vi "Teleop.vi"(10 "Match Info":T1={"Autonomous Elapsed Seconds"=0.0, "TeleOp Elapsed Seconds"=0.0, "Disabled Elapsed Seconds"=0.0, "Visited Autonomous"=FALSE, "Visited TeleOp"=FALSE, "Visited Disabled"=FALSE, "Autonomous Settings"={"Autonomous Style"=enum."Independent", "VI Refnum"=refnum}}, 11 "Call Context":T2) -> ()   [LabVIEW 2020]
doc: "This VI is called for each TeleOp packet received from the DS where the robot is not disabled. It is often used to read from the joysticks and update I/O or to update setpoints for timed control loops. It should complete and return within 20 milliseconds or it may miss DS packets."
uses:
  <vilib>/Rock Robotics/WPI/DriverStation/WPI_DriverStationDerivedRobotMode.ctl
  <vilib>/Rock Robotics/WPI/DriverStation/WPI_DriverStationMatch Info.ctl
  <vilib>/Rock Robotics/WPI/ThirdParty/Phoenix-LabVIEW/Motor Controller/Controls/CTRE_Phoenix_MotorControl_ControlMode.ctl
  <vilib>/Rock Robotics/Network Tables/NT Read Boolean.vi
  <vilib>/Rock Robotics/Network Tables/NT Read Number.vi
  <vilib>/Rock Robotics/WPI/Utilities/WPI_GetSetVariantRefNum.vi
  <vilib>/Rock Robotics/WPI/ThirdParty/Phoenix-LabVIEW/Motor Controller/Get/CTRE_Phoenix_MotorController_GetSelectedSensorData.vi
panel:
  out "Angle Back Left":dbl
  out "Angle Back Right":dbl
  out "Angle Front Right":dbl
  out "Angle Front Left":dbl
  out "Speed Back Left":dbl
  out "Speed Back Right":dbl
  out "Speed Front Right":dbl
  out "Speed Front Left":dbl
  in  "reverse steer":bool=TRUE
  in  "reverse encoder":bool=TRUE
  in  "ScaleSpeed":dbl=1.0
  in  "upper limit":dbl=0.02
  in  "lower limit":dbl=-0.02
  in  "Wheelbase":dbl=23.75
  in  "Trackwidth":dbl=18.1
  out "Sample Slider 0":dbl(slide) scale=0.0..5.0
  out "Sample Boolean 1":bool
  out "Sample Boolean 0":bool
  # "This column has configuration\nconstants for the swerve\ndrives. ReverseSteer and \nRevereEncoder should stay\n\"on\" (true) unless your hardware\nrequires it to be set otherwise."
  # "This column is debug \noutput for the 4 swerve\ndrives - wheel speed and \nangle info."
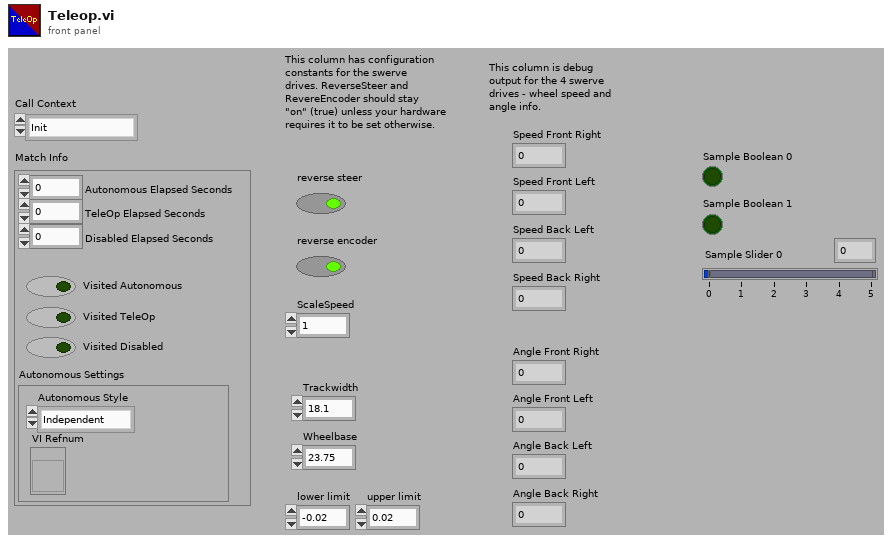
[diagram p1: front panel]
types:
  T1 = typedef "WPI_DriverStationMatch Info.ctl" = cluster{"Autonomous Elapsed Seconds":dbl, "TeleOp Elapsed Seconds":dbl, "Disabled Elapsed Seconds":dbl, "Visited Autonomous":bool, "Visited TeleOp":bool, "Visited Disabled":bool, "Autonomous Settings":cluster{"Autonomous Style":enum16{"Iterative", "Independent"}, "VI Refnum":refnum<vi>}}
  T2 = typedef "WPI_DriverStationDerivedRobotMode.ctl" = enum16{"Init", "Execute", "Stop"}
  T3 = typedef "CTRE_Phoenix_MotorControl_ControlMode.ctl" = u16
  T4 = typedef "WPI_JoystickDevRef.ctl" = cluster{"Device":T5}
  T5 = typedef "WPI_JoystickDeviceEnum.ctl" = enum16{"USB 0", "USB 1", "USB 2", "USB 3", "USB 4", "USB 5"}
  T6 = typedef "WPI_MotorControlDeviceRef.ctl" = cluster{"DeviceStatus":errorcluster, "Type":T7, "PWM":cluster{"PWM Channel":T8, "DeadBand":T9}, "CAN":cluster{"Device Number":u8, "SetOutput VI Ref":variant, "GetOutput VI Ref":variant, "Enable VI Ref":variant, "Disable VI Ref":variant, "Data":variant}, "Invert":bool, "DIO PWM":cluster{"PWM \"Enable\" Channel":T8, "DIOChannel":T10, "PWM Rate":dbl}}
  T7 = typedef "WPI_MotorControlType.ctl" = enum16{"PWM", "CAN", "DIO PWM"}
  T8 = typedef "FPGA_DIOPWMChannel.ctl" = enum8{"PWM 0", "PWM 1", "PWM 2", "PWM 3", "PWM 4", "PWM 5", "PWM 6", "PWM 7", "PWM 8", "PWM 9", "PWM MXP 0", "PWM MXP 1", "PWM MXP 2", "PWM MXP 3", "PWM MXP 4", "PWM MXP 5", "PWM MXP 6", "PWM MXP 7", "PWM MXP 8", "PWM MXP 9", "Invalid"}
  T9 = typedef "WPI_PWMDeadband.ctl" = cluster{"Name":string, "maxPositivePwm":i32, "minPositivePwm":i32, "centerPwm":i32, "maxNegativePwm":i32, "minNegativePwm":i32, "angularRange":u16}
  T10 = typedef "FPGA_DIOChannel.ctl" = enum8{"DIO 0", "DIO 1", "DIO 2", "DIO 3", "DIO 4", "DIO 5", "DIO 6", "DIO 7", "DIO 8", "DIO 9", "DIO MXP 0", "DIO MXP 1", "DIO MXP 2", "DIO MXP 3", "DIO MXP 4", "DIO MXP 5", "DIO MXP 6", "DIO MXP 7", "DIO MXP 8", "DIO MXP 9", "DIO MXP 10", "DIO MXP 11", "DIO MXP 12", "DIO MXP 13", "DIO MXP 14", "DIO MXP 15", "SPI Port CS1", "SPI Port CS2", "SPI Port CS3", "SPI Port MISO", "SPI Port MOSI", "Invalid"}
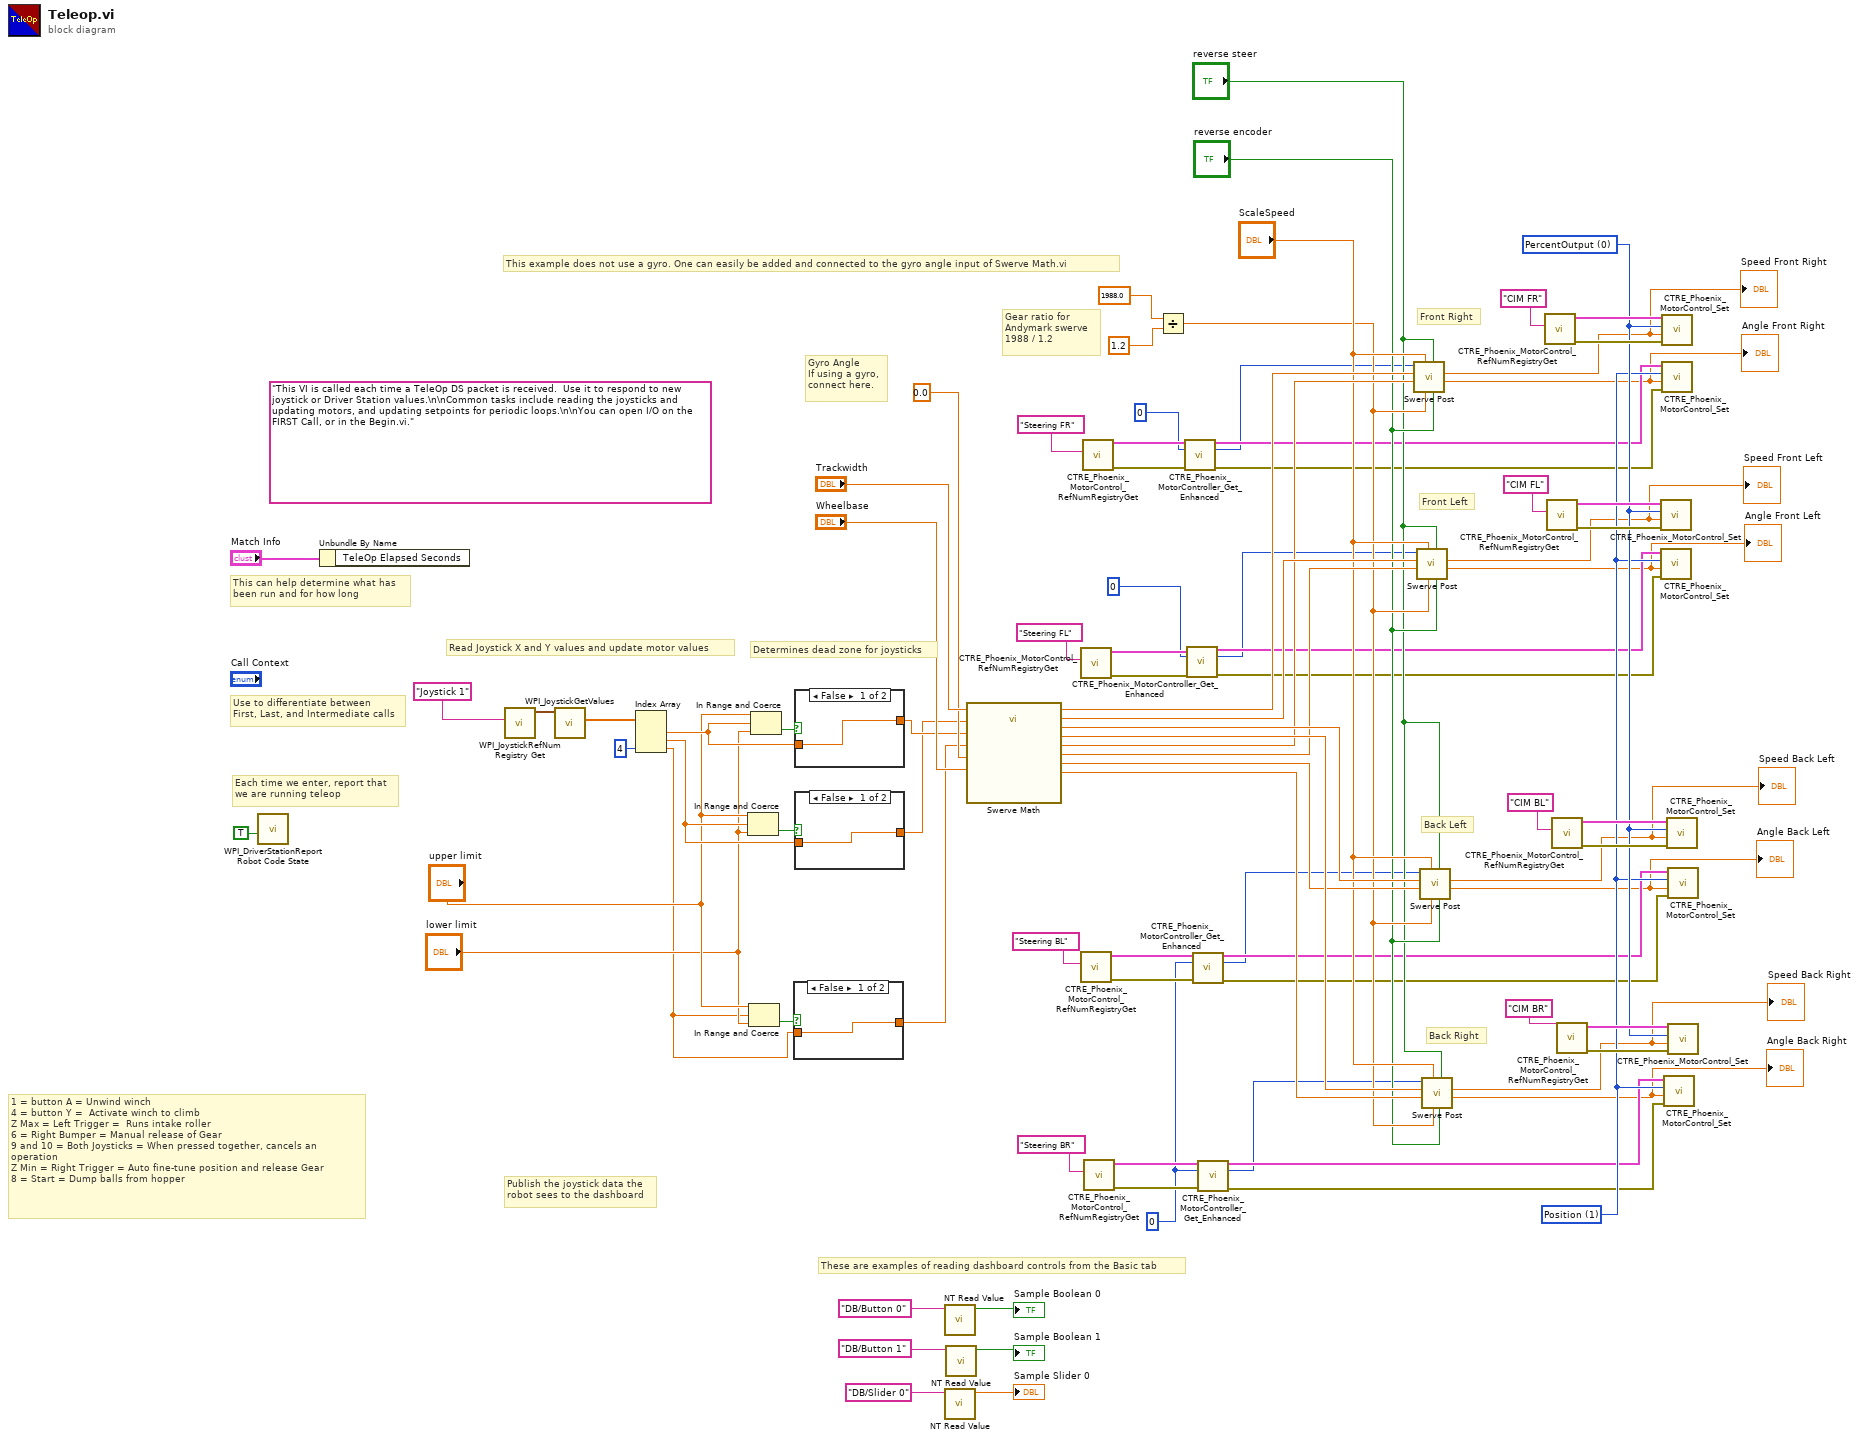
[diagram p0: block diagram]
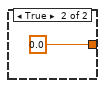
[diagram p2: hidden frame]
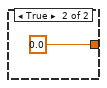
[diagram p3: hidden frame]
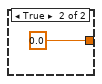
[diagram p4: hidden frame]
diagram:
  w26 = u32 0 ("pidLoopIdx")
  w35 = T3 1 items=["PercentOutput"=0, "Position"=1, "Velocity"=2, "Current"=3, "Follower"=5, "MotionProfile"=6, "MotionMagic"=7, "MotionProfileArc"=10, "Disabled"=15] ("Control Mode")
  w36 = T3 0 items=["PercentOutput"=0, "Position"=1, "Velocity"=2, "Current"=3, "Follower"=5, "MotionProfile"=6, "MotionMagic"=7, "MotionProfileArc"=10, "Disabled"=15] ("Control Mode")
  (unwired) "This VI is called each time a TeleOp DS packet is received.  Use it to respond to new joystick or Driver Station values.\n\nCommon tasks include reading the joysticks and updating motors, and updating setpoints for periodic loops.\n\nYou can open I/O on the FIRST Call, or in the Begin.vi."
  # "Gear ratio for\nAndymark swerve\n1988 / 1.2"
  # "Back Right"
  # "Back Left"
  # "Front Left"
  # "Front Right"
  # "This example does not use a gyro. One can easily be added and connected to the gyro angle input of Swerve Math.vi"
  # "1 = button A =\tUnwind winch\n4 = button Y = \tActivate winch to climb\nZ Max = Left Trigger = \tRuns intake roller\n6 = Right Bumper = Manual release of Gear\n9 and 10 = Both Joysticks = When pressed together, cancels an operation\nZ Min = Right Trigger = Auto fine-tune position and release Gear \n8 = Start = Dump balls from hopper"
  # "Determines dead zone for joysticks"
  # "Gyro Angle\nIf using a gyro,\nconnect here."
  # "Publish the joystick data the\nrobot sees to the dashboard"
  # "These are examples of reading dashboard controls from the Basic tab"
  # "Each time we enter, report that\nwe are running teleop"
  # "Use to differentiate between\nFirst, Last, and Intermediate calls"
  # "This can help determine what has\nbeen run and for how long"
  # "Read Joystick X and Y values and update motor values"
  n1 = call <vilib>:"WPI_DriverStationReport Robot Code State.vi"("TeleOp"=TRUE ("Autonomous")) -> ()  [unwired: 10 in, 1 out]
  n2 = Unbundle By Name("Match Info") -> ()  [unwired: 1 out]
  n3 = call <vilib>:"WPI_JoystickRefNum Registry Get.vi"("refnum name"="Joystick 1") -> ("JoystickDevRef"=w80:T4)  [unwired: 1 in, 9 out]
  n4 = call <vilib>:"WPI_JoystickGetValues.vi"("JoystickDevRef"=w80) -> ("Axes"=w79:dbl[])  [unwired: 6 in, 4 out]
  n5 = Index Array(array=w79, index #3=4 ("index")) -> (element #1=w60:dbl, element #2=w61:dbl, element #3=w4:dbl)  [unwired: 2 in]
  n6 = In Range and Coerce(upper limit="upper limit", x=w61, lower limit="lower limit") -> (In Range?=w66:bool)  [unwired: 1 out]
  n7 = In Range and Coerce(upper limit="upper limit", x=w4, lower limit="lower limit") -> (In Range?=w67:bool)  [unwired: 1 out]
  n8 = In Range and Coerce(upper limit="upper limit", x=w60, lower limit="lower limit") -> (In Range?=w65:bool)  [unwired: 1 out]
  n9 = case shown="False" w67 {
    tunnel: [w90 0.0 ("Gyro Angle")] -> w64
    tunnel: w4 -> [w90 _]
    frame False {
    }
    frame True {
    }
  }
  n10 = case shown="False" w65 {
    tunnel: [w92 0.0 ("Gyro Angle")] -> w63
    tunnel: w60 -> [w92 _]
    frame False {
    }
    frame True {
    }
  }
  n11 = case shown="False" w66 {
    tunnel: [w94 0.0 ("Gyro Angle")] -> w62
    tunnel: w61 -> [w94 _]
    frame False {
    }
    frame True {
    }
  }
  n12 = call-poly <vilib>:"NT Read Value.vi"("Name"="DB/Button 0" ("refnum name")) -> ("Boolean"=→"Sample Boolean 0":bool)  [unwired: 9 in, 1 out]
  n13 = call-poly <vilib>:"NT Read Value.vi"("Name"="DB/Slider 0" ("refnum name")) -> ("Numeric"=→"Sample Slider 0":dbl)  [unwired: 9 in, 1 out]
  n14 = call-poly <vilib>:"NT Read Value.vi"("Name"="DB/Button 1" ("refnum name")) -> ("Boolean"=→"Sample Boolean 1":bool)  [unwired: 9 in, 1 out]
  n15 = call "Swerve Math.vi"("Trackwidth (W)"="Trackwidth", "Wheelbase (L)"="Wheelbase", "Y -FWD"=w62, "X1 STR"=w63, "X2 RCW"=w64, "Gyro Angle in degrees"=0.0 ("Gyro Angle")) -> ("wa3"=w51:dbl, "wa4"=w50:dbl, "FR Speed"=w56:dbl, "FL Speed"=w55:dbl, "BL Speed"=w54:dbl, "BR Speed"=w57:dbl, "wa2"=w52:dbl, "wa1"=w53:dbl)  [unwired: 2 in]
  n16 = call <vilib>:"CTRE_Phoenix_MotorControl_RefNumRegistryGet.vi"("refnum name"="Steering FL") -> ("error out"=w21:errorcluster, "PhoenixMotorControlDevRef"=w22:T6)  [unwired: 9 in]
  n17 = call <vilib>:"CTRE_Phoenix_MotorControl_RefNumRegistryGet.vi"("refnum name"="Steering BL") -> ("error out"=w30:errorcluster, "PhoenixMotorControlDevRef"=w31:T6)  [unwired: 9 in]
  n18 = call <vilib>:"CTRE_Phoenix_MotorControl_RefNumRegistryGet.vi"("refnum name"="Steering FR") -> ("error out"=w16:errorcluster, "PhoenixMotorControlDevRef"=w17:T6)  [unwired: 9 in]
  n19 = call <vilib>:"CTRE_Phoenix_MotorControl_RefNumRegistryGet.vi"("refnum name"="Steering BR") -> ("error out"=w32:errorcluster, "PhoenixMotorControlDevRef"=w33:T6)  [unwired: 9 in]
  n20 = Divide(x=1988.0, y=1.2) -> (x/y=w46:dbl)
  n21 = call-poly <vilib>:"CTRE_Phoenix_MotorController_Get_Enhanced.vi"("PhoenixMotorControlDevRef"=w17, "pidLoopIdx"=u32 0, "error in"=w16) -> ("PhoenixMotorControlDevRef"=w14:T6, "Position (Raw Sensor Units)"=w13:i32, "error out"=w15:errorcluster)  [unwired: 9 in, 1 out]
  n22 = call-poly <vilib>:"CTRE_Phoenix_MotorController_Get_Enhanced.vi"("PhoenixMotorControlDevRef"=w22, "pidLoopIdx"=u32 0, "error in"=w21) -> ("PhoenixMotorControlDevRef"=w19:T6, "Position (Raw Sensor Units)"=w18:i32, "error out"=w20:errorcluster)  [unwired: 9 in, 1 out]
  n23 = call-poly <vilib>:"CTRE_Phoenix_MotorController_Get_Enhanced.vi"("PhoenixMotorControlDevRef"=w31, "pidLoopIdx"=w26, "error in"=w30) -> ("PhoenixMotorControlDevRef"=w28:T6, "Position (Raw Sensor Units)"=w27:i32, "error out"=w29:errorcluster)  [unwired: 9 in, 1 out]
  n24 = call-poly <vilib>:"CTRE_Phoenix_MotorController_Get_Enhanced.vi"("PhoenixMotorControlDevRef"=w33, "pidLoopIdx"=w26, "error in"=w32) -> ("PhoenixMotorControlDevRef"=w24:T6, "Position (Raw Sensor Units)"=w23:i32, "error out"=w25:errorcluster)  [unwired: 9 in, 1 out]
  n25 = call "Swerve Post.vi"("reverse encoder"="reverse encoder", "reverse steer"="reverse steer", "gear ratio"=w46, "ScaleSpeed"="ScaleSpeed", "wa in"=w53, "ws in"=w56, "encoder in"=w13) -> ("wa out"=w6:dbl, "ws out 0-1"=w5:dbl)  [unwired: 3 in]
  "Speed Front Right" <- w5
  "Angle Front Right" <- w6
  n26 = call "Swerve Post.vi"("reverse encoder"="reverse encoder", "reverse steer"="reverse steer", "gear ratio"=w46, "ScaleSpeed"="ScaleSpeed", "wa in"=w52, "ws in"=w55, "encoder in"=w18) -> ("wa out"=w8:dbl, "ws out 0-1"=w7:dbl)  [unwired: 3 in]
  "Speed Front Left" <- w7
  "Angle Front Left" <- w8
  n27 = call "Swerve Post.vi"("reverse encoder"="reverse encoder", "reverse steer"="reverse steer", "gear ratio"=w46, "ScaleSpeed"="ScaleSpeed", "wa in"=w51, "ws in"=w54, "encoder in"=w27) -> ("wa out"=w10:dbl, "ws out 0-1"=w9:dbl)  [unwired: 3 in]
  "Speed Back Left" <- w9
  "Angle Back Left" <- w10
  n28 = call "Swerve Post.vi"("reverse encoder"="reverse encoder", "reverse steer"="reverse steer", "gear ratio"=w46, "ScaleSpeed"="ScaleSpeed", "wa in"=w50, "ws in"=w57, "encoder in"=w23) -> ("wa out"=w12:dbl, "ws out 0-1"=w11:dbl)  [unwired: 3 in]
  "Speed Back Right" <- w11
  "Angle Back Right" <- w12
  n29 = call <vilib>:"CTRE_Phoenix_MotorControl_RefNumRegistryGet.vi"("refnum name"="CIM FR") -> ("error out"=w43:errorcluster, "PhoenixMotorControlDevRef"=w44:T6)  [unwired: 9 in]
  n30 = call <vilib>:"CTRE_Phoenix_MotorControl_RefNumRegistryGet.vi"("refnum name"="CIM FL") -> ("error out"=w41:errorcluster, "PhoenixMotorControlDevRef"=w42:T6)  [unwired: 9 in]
  n31 = call <vilib>:"CTRE_Phoenix_MotorControl_RefNumRegistryGet.vi"("refnum name"="CIM BL") -> ("error out"=w39:errorcluster, "PhoenixMotorControlDevRef"=w40:T6)  [unwired: 9 in]
  n32 = call <vilib>:"CTRE_Phoenix_MotorControl_RefNumRegistryGet.vi"("refnum name"="CIM BR") -> ("error out"=w37:errorcluster, "PhoenixMotorControlDevRef"=w38:T6)  [unwired: 9 in]
  n33 = call <vilib>:"CTRE_Phoenix_MotorControl_Set.vi"("error in (no error)"=w41, "Output"=w7, "Control Mode"=w36, "PhoenixMotorControlDevRef"=w42) -> ()  [unwired: 6 in, 2 out]
  n34 = call <vilib>:"CTRE_Phoenix_MotorControl_Set.vi"("error in (no error)"=w20, "Output"=w8, "Control Mode"=w35, "PhoenixMotorControlDevRef"=w19) -> ()  [unwired: 6 in, 2 out]
  n35 = call <vilib>:"CTRE_Phoenix_MotorControl_Set.vi"("error in (no error)"=w43, "Output"=w5, "Control Mode"=w36, "PhoenixMotorControlDevRef"=w44) -> ()  [unwired: 6 in, 2 out]
  n36 = call <vilib>:"CTRE_Phoenix_MotorControl_Set.vi"("error in (no error)"=w15, "Output"=w6, "Control Mode"=w35, "PhoenixMotorControlDevRef"=w14) -> ()  [unwired: 6 in, 2 out]
  n37 = call <vilib>:"CTRE_Phoenix_MotorControl_Set.vi"("error in (no error)"=w25, "Output"=w12, "Control Mode"=w35, "PhoenixMotorControlDevRef"=w24) -> ()  [unwired: 6 in, 2 out]
  n38 = call <vilib>:"CTRE_Phoenix_MotorControl_Set.vi"("error in (no error)"=w39, "Output"=w9, "Control Mode"=w36, "PhoenixMotorControlDevRef"=w40) -> ()  [unwired: 6 in, 2 out]
  n39 = call <vilib>:"CTRE_Phoenix_MotorControl_Set.vi"("error in (no error)"=w29, "Output"=w10, "Control Mode"=w35, "PhoenixMotorControlDevRef"=w28) -> ()  [unwired: 6 in, 2 out]
  n40 = call <vilib>:"CTRE_Phoenix_MotorControl_Set.vi"("error in (no error)"=w37, "Output"=w11, "Control Mode"=w36, "PhoenixMotorControlDevRef"=w38) -> ()  [unwired: 6 in, 2 out]
